vi "POST.vi"(8 "error in (no error)":errorcluster, 9 "timeout (10000)":i32=10000, 10 "Request String":string, 11 "url":string) -> (0 "error out":errorcluster, 3 "JSON Value out":refnum<class "JSON Value.lvclass">)   [LabVIEW 2021]
uses:
  <vilib>/NI/JSON Support for LabVIEW/JSON Value/JSON Value.lvclass
  <vilib>/httpClient/POSTBuffer.vi
  <vilib>/httpClient/LabVIEWHTTPClient.lvlib
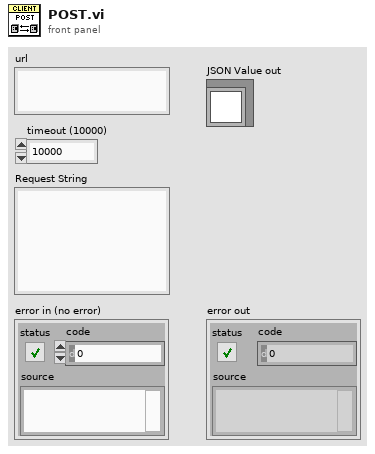
[diagram p1: front panel]
types:
  T1 = typedef "LabVIEWHTTPClient.lvlib/ClientHandle.ctl" = refnum<k1>
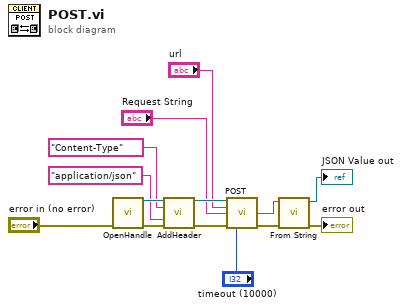
[diagram p0: block diagram]
diagram:
  n1 = call <vilib>:"OpenHandle.vi"("error in (no error)"="error in (no error)") -> ("client handle out"=w8:T1, "error out"=w10:errorcluster)  [unwired: 13 in]
  n2 = call <vilib>:"AddHeader.vi"("client handle"=w8, "header"="Content-Type", "value"="application/json" ("header value"), "error in (no error)"=w10) -> ("client handle out"=w5:T1, "error out"=w4:errorcluster)  [unwired: 10 in]
  n3 = call-poly <vilib>:"POST.vi"("client handle"=w5, "url"="url", "buffer"="Request String", "error in (no error)"=w4, "timeout (10000)"="timeout (10000)") -> ("body"=w13:string, "error out"=w11:errorcluster)  [unwired: 7 in, 2 out]
  n4 = call <vilib>:"From String.vi"("error in (no error)"=w11, "JSON String"=w13) -> ("error out"=→"error out":errorcluster, "JSON Value out"=→"JSON Value out":refnum<class "JSON Value.lvclass">)  [unwired: 8 in]
